vi "CameraSetScaledAttrSharpness.vi"(6 "Exposure Fixup?":bool, 8 "error in (no error)":errorcluster, 9 "Scaled":dbl, 10 "Attr String":string, 11 "IMAQdx Session":T1) -> (0 "error out":errorcluster, 3 "IMAQdx Session out":T1)   [LabVIEW 2025]
doc: "This VI updates an attribute where input unit is percentage and camera parameter may be in another unit.\n\nThis software is licensed. Open the labview\\readme\\WPI Robotics Library Open Source License.txt file for more information."
uses:
  <vilib>/userDefined/High Color/IMAQdx.ctl
  <resource>/objmgr/imaqdx.rc
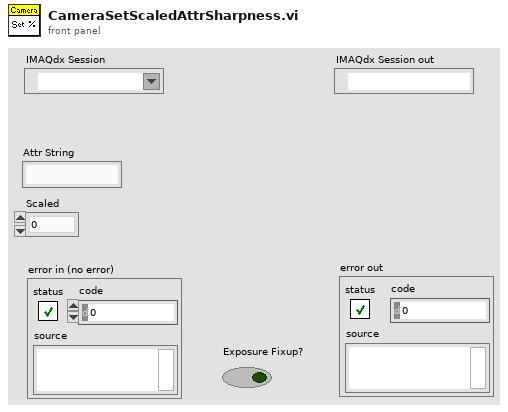
[diagram p1: front panel]
types:
  T1 = typedef "IMAQdx.ctl" = refnum<k21>
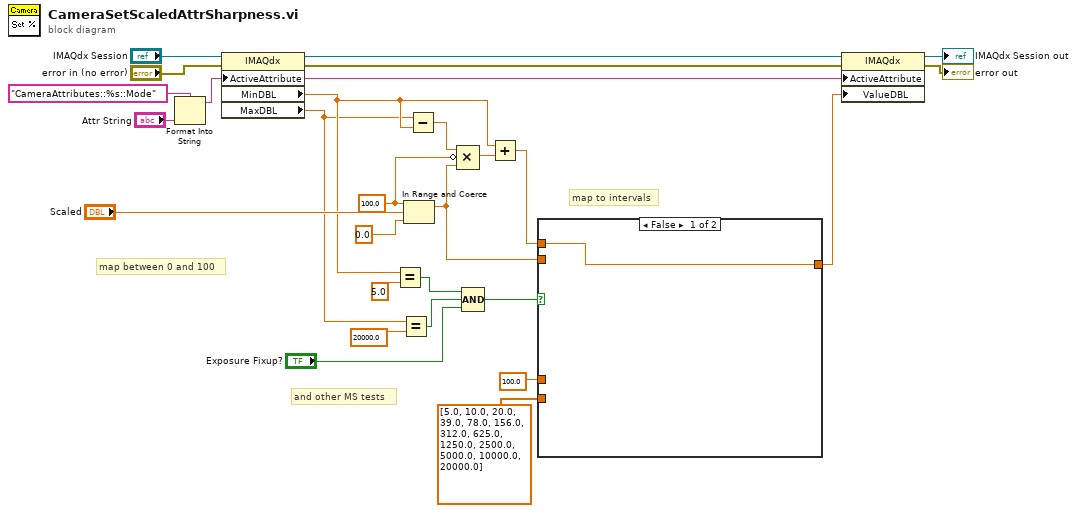
[diagram p0: block diagram]
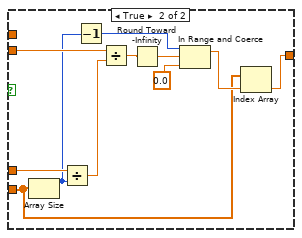
[diagram p2: hidden frame]
diagram:
  w24 = 100.0
  # "map to intervals"
  # "and other MS tests"
  # "map between 0 and 100"
  n1 = Format Into String(format string="CameraAttributes::%s::Mode" ("Attr Format"), "Attr String") -> (resulting string=w1:string)  [unwired: 2 in, 1 out]
  n2 = property class="IMAQdx"(reference="IMAQdx Session", error in="error in (no error)", "ActiveAttribute"=w1) -> (reference out=w22:T1, error out=w20:errorcluster, "MinDBL"=w18:dbl, "MaxDBL"=w15:dbl)
  n3 = Equal?(x=w18, y=5.0) -> (x = y?=w14:bool)
  n4 = Equal?(x=w15, y=20000.0) -> (x = y?=w13:bool)
  n5 = In Range and Coerce(upper limit=w24, x="Scaled", lower limit=0.0) -> (coerced(x)=w11:dbl)  [unwired: 1 out]
  n6 = Subtract(x=w15, y=w18) -> (x-y=w27:dbl)
  n7 = Compound Arithmetic op=MULTIPLY(w27, invert w24, w11) -> (w23:dbl)
  n8 = Compound Arithmetic op=AND(w14, w13, "Exposure Fixup?") -> (w12:bool)
  n9 = Add(x=w18, y=w23) -> (x+y=w8:dbl)
  n10 = case shown="False" w12 {
    tunnel: w8 -> [w28 _]
    tunnel: w11 -> [_ w39]
    tunnel: dbl[] [5.0, 10.0, 20.0, 39.0, 78.0, 156.0, 312.0, 625.0, 1250.0, 2500.0, 5000.0, 10000.0, 20000.0] -> [_ w31]
    tunnel: 100.0 -> [_ w38]
    tunnel: [w28 w37] -> w7
    frame False {
    }
    frame True {
      n11 = Array Size(array=w31) -> (size(s)=w29:i32)
      n12 = Divide(x=w38, y=w29) -> (x/y=w36:dbl)
      n13 = Decrement(x=w29) -> (x-1=w30:i32)
      n14 = Divide(x=w39, y=w36) -> (x/y=w35:dbl)
      n15 = Round Toward -Infinity(1:w35) -> (0:w34:dbl)
      n16 = In Range and Coerce(upper limit=w30, x=w34, lower limit=0.0) -> (coerced(x)=w33:dbl)  [unwired: 1 out]
      n17 = Index Array(array=w31, index=w33) -> (element=w37:dbl)
    }
  }
  n18 = property class="IMAQdx"(reference=w22, error in=w20, "ActiveAttribute"=w1, "ValueDBL"=w7) -> (reference out=→"IMAQdx Session out":T1, error out=→"error out":errorcluster)
